vi "HFRR ADV v04.vi"() -> ()   [LabVIEW 2025] (continued)
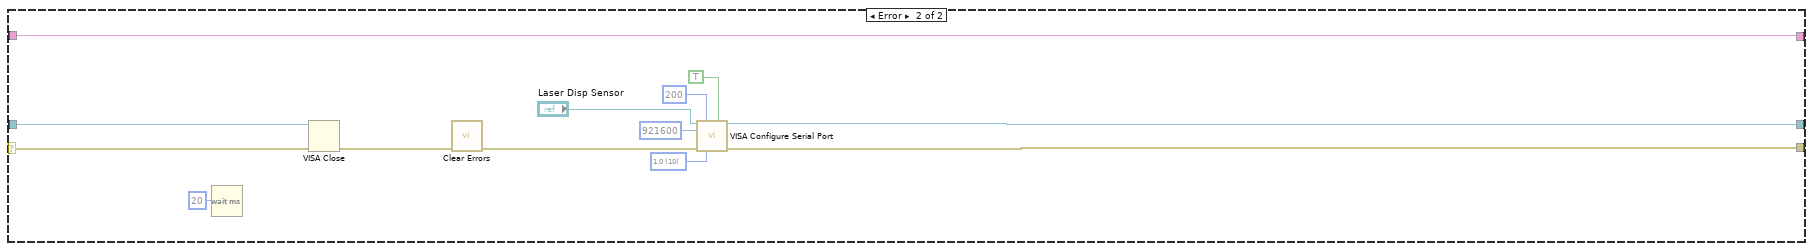
[diagram p11: hidden frame]
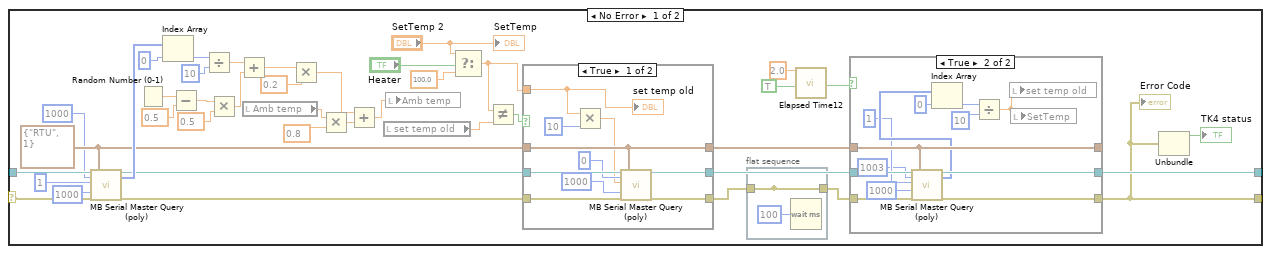
[diagram p13: hidden frame]
            n2851 = Concatenate Strings(w3863, w3862, w3864) -> (w3861:string)
            n2852 = Concatenate Strings(w3860, w3872, w3889, w3830) -> (w3836:string)
            n2853 = Concatenate Strings(w3860, w3871, w3882, w3830) -> (w3835:string)
            n2854 = Concatenate Strings(w3860, w3870, w3881, w3830) -> (w3834:string)
            n2855 = Concatenate Strings(w3860, w3869, w3874, w3830) -> (w3833:string)
            n2856 = Concatenate Strings(w3860, w3859, w3868, w3830) -> (w3832:string)
            n2857 = Concatenate Strings(w3860, w3858, w3861, "\"}" ("string")) -> (w3831:string)
            n2858 = Concatenate Strings(w3837, w3836, w3835, w3834, w3833, w3832, w3831, "]}" ("string")) -> (w3828:string)
            n2859 = local read "SEN.RUN HRS"() -> (w3795:dbl)
            n2860 = disable-structure shown="Disabled" {
              frame Disabled {
                n2861 = local read "state"() -> (w3914:string[])
                n2862 = Delete From Array(array=w3914, index=0) -> (array with subset deleted=w3912:string[])  [unwired: 1 in, 1 out]
                n2863 = for {
                  N: 6 -> [_]
                  tunnel: w3912 -> [w3925] mode=indexing
                  tunnel: [w3924] -> w3911 mode=indexing
                  n2864 = Equal?(x=w3925, y="Warning") -> (x = y?=w3921:bool)
                  n2865 = Equal?(x=w3925, y="Healthy") -> (x = y?=w3918:bool)
                  n2866 = Select(t="2" ("y"), s=w3921, f="3" ("y")) -> (s? t:f=w3916:string)
                  n2867 = Select(t="1" ("y"), s=w3918, f=w3916) -> (s? t:f=w3924:string)
                }
                "state1" <- w3911
              }
              frame Enabled {
              }
            }
            n2868 = stacked-sequence {
              tunnel: w3828 -> [w3936 _ _]
              tunnel: [_ _ w3952] -> _
              frame #0 {
                (unwired) FALSE ("convert eol (F)")
                w3938 = enum16{"start", "end", "current"}."start" ("pos mode (0:2)")
                n2869 = local read "Path"() -> (w3932:path)
                n2870 = Path To String(path=w3932) -> (string=w3944:string)
                n2871 = Concatenate Strings(w3944, "\\", "Sensor File Name") -> (w3945:string)
                n2872 = local write "standard output 2"(" ") -> ()
                n2873 = String To Path(string=w3945) -> (path=w3935:path)
                n2874 = call <vilib>:"Open_Create_Replace File.vi"("advisory dialog? (display:T)"=FALSE, "function (open:0)"=T22."create or replace", "file path"=w3935) -> ("error out"=w3948:errorcluster, "refnum"=w3947:refnum<file>)  [unwired: 5 in, 2 out]
                n2875 = Set File Position(refnum=w3947, from (0:start)=w3938, error in=w3948) -> (refnum out=w3928:refnum<file>, error out=w3927:errorcluster)  [unwired: 1 in]
                n2876 = Write to Binary File(file (use dialog)=w3928, data=" ", error in=w3927, 5:FALSE ("prepend array or string size? (T)")) -> (refnum out=w3939:refnum<file>, error out=w3940:errorcluster)  [unwired: 2 in, 1 out]
                n2877 = Set File Position(offset (in bytes) (0)=w3938, refnum=w3939, error in=w3940) -> (refnum out=w3931:refnum<file>, error out=w3930:errorcluster)  [unwired: 1 in]
                n2878 = Write to Binary File(file (use dialog)=w3931, data=w3936, error in=w3930, 5:FALSE ("prepend array or string size? (T)")) -> (error out=w3934:errorcluster)  [unwired: 2 in, 2 out]
                n2879 = flat-sequence {
                  tunnel: w3935 -> [w3950]
                  tunnel: w3934 -> [_]
                  frame #0 {
                    n2880 = call <vilib>:"Read Characters From File.vi"("file path (dialog if empty)"=w3950) -> ("character string"=→"Sensor Health JSON string":string)  [unwired: 5 in, 3 out]
                  }
                }
                "SinglePoint  2" <- w3936
              }
              frame #1 {
              }
              frame #2 {
                (unwired) "\"Stored\": true" ("string")
                n2881 = call <vilib>:"System Exec.vi"("run minimized? (F)"=TRUE, "wait until completion? (T)"=TRUE, "working directory"=path "C:/LAB-IQ-NXT", "command line"="C:\\LAB-IQ-NXT\\JPostH.bat") -> ("standard error"=→"Respose From Server 2":string, "standard output"=w3955:string)  [unwired: 4 in, 2 out]
                "standard output 2" <- w3955
                n2882 = Match Pattern(string=w3955, regular expression="JSONH Check String") -> (match substring=w3953:string, offset past match=w3952:i32)  [unwired: 1 in, 2 out]
                n2883 = Equal?(x=w3953, y="JSONH Check String") -> (x = y?=→"Upload \nConfirmed 2":bool)
              }
            }
            n2884 = Divide(x=w3795, y=3600.0 ("f")) -> (x/y=w3788:dbl)
            n2885 = local read "run time"() -> (w3845:string[])
            n2886 = Round To Nearest(number=w3788) -> (nearest integer value=w3787:dbl)
            n2887 = Number To Decimal String(number=w3787) -> (decimal integer string=w3786:string)  [unwired: 1 in]
            n2888 = Index Array(array="Sensor Information", index (col) #1=0 ("disabled index (col)"), index (col) #2=1 ("index (col)"), index (col) #3=2 ("index (col)"), index (col) #4=3 ("index (col)")) -> (element #1=→"Sensor name":string[], element #2=→"model num":string[], element #3=→"run time":string[], element #4=→"state":string[])  [unwired: 4 in]
            n2889 = Insert Into Array(array=w3845, index=1, new element #1=w3786, new element #2=w3786, new element #3=w3786, new element #4=w3786, new element #5=w3786, new element #6=w3786) -> (w3810:string[])
            "run" <- w3810
            n2890 = local read "out"() -> (w3792:string[])
            n2891 = local read "Sensor Information"() -> (w3812:string[][])
            n2892 = Replace Array Subset(array=w3812, new element #1=w3810, index (col) #1=2 ("disabled index (col)"), new element #2=w3792, index (col) #2=3 ("index (col)")) -> (w3811:string[][])  [unwired: 2 in]
            n2893 = local write "Sensor Information"(w3811) -> ()
          }
        }
        n2894 = case shown="True" w3759 {
          frame False {
          }
          frame True {
            n2895 = Equal?(x="FLAG", y=0.0) -> (x = y?=w3776:bool)
            n2896 = case shown="False" w3776 {
              frame False {
                n2897 = Get Date/Time In Seconds() -> (seconds since 1Jan1904=w3782:timestamp)
                n2898 = local read "START 2"() -> (w3780:dbl)
                n2899 = To Double Precision Float(number=w3782) -> (double precision float=w3781:dbl)
                n2900 = Subtract(x=w3781, y=w3780) -> (x-y=→"SENSOR TIME  2":dbl)
              }
              frame True {
                n2901 = Get Date/Time In Seconds() -> (seconds since 1Jan1904=w3784:timestamp)
                n2902 = To Double Precision Float(number=w3784) -> (double precision float=→"START 2":dbl)
                n2903 = local write "FLAG"(100.0 ("FLAG")) -> ()
              }
            }
          }
        }
        n2904 = disable-structure shown="Disabled" {
          disable-tunnel: w3762 -> [w3771 _]
          disable-tunnel: [w3770 _] -> w3761
          frame Disabled {
            n2905 = local read "Json St Flg"() -> (w3769:bool)
            n2906 = case shown="True" w3769 {
              tunnel: w3771 -> [w3772 w3774]
              tunnel: [w3772 w3773] -> w3770
              frame False {
              }
              frame True {
                n2907 = Increment(x=w3774) -> (x+1=w3773:dbl)
                "T cycle" <- w3773
                n2908 = local write "Json St Flg"(FALSE ("Json St Flg")) -> ()
              }
            }
          }
          frame Enabled {
          }
        }
        n2909 = local read "EXIT"() -> (w3756:bool)
      }
    }
    frame Enabled {
    }
  }
  n2910 = stacked-sequence {
    tunnel: [w4154] -> w16
    frame #0 {
      w4154 = FALSE ("Upload \nConfirmed")
      n2911 = local write "Upload \nConfirmed"(w4154) -> ()
      n2912 = local write "St Str"("") -> ()
    }
  }
  n2913 = disable-structure shown="Disabled" {
    disable-tunnel: w16 -> [w4155 _]
    frame Disabled {
      n2914 = case shown="True" {
        selector: _ -> [_ _]
        tunnel: w4155 -> [_ w4156]
        frame False {
        }
        frame True {
          n2915 = while {
            tunnel: [w4162] -> _
            tunnel: w4156 -> [_]
            i -> [w4162]
            stop <- w4159 stop-if-true
            n2916 = local read "Json End Flg"() -> (w4161:bool)
            n2917 = Wait (ms)(milliseconds to wait=u32 20 ("Refresh Rate (ms)")) -> ()  [unwired: 1 out]
            n2918 = local read "refresh flag"() -> (w4157:bool)
            n2919 = local read "RUN"() -> (w4158:bool)
            n2920 = And(x=w4158, y=w4157) -> (x .and. y?=w4160:bool)
            n2921 = Or(x=w4160, y=w4161) -> (x .or. y?=w4163:bool)
            "AR Led" <- w4163
            n2922 = case shown="True" w4163 {
              frame False {
              }
              frame True {
                w4180 = "\",\""
                n2923 = local read "UUID"() -> (w4178:string)
                n2924 = local write "refresh flag"(FALSE ("refresh flag")) -> ()
                n2925 = local read "time"() -> (w4167:dbl)
                n2926 = Multiply(x=w4167, y=60.0) -> (x*y=w4166:dbl)
                n2927 = Concatenate Strings("UUID\" : \"", w4178, "\"}") -> (w4181:string)
                n2928 = Number To Fractional String(number=w4166, width (-)=i16 10, precision (6)=i16 4) -> (F-format string=w4195:string)  [unwired: 1 in]
                n2929 = Concatenate Strings("{", "\"Time\":\"", w4195, w4180) -> (w4190:string)
                n2930 = stacked-sequence {
                  tunnel: w4180 -> [w4243 w4251 w4258 w4266 w4274 w4283 w4290]
                  tunnel: [w4244 _ _ _ _ _ _] -> w4194
                  tunnel: [_ w4252 _ _ _ _ _] -> w4193
                  tunnel: [_ _ w4259 _ _ _ _] -> w4192
                  tunnel: [_ _ _ w4268 _ _ _] -> w4191
                  tunnel: w4181 -> [_ _ _ _ _ _ w4301]
                  tunnel: [_ _ _ _ _ _ w4300] -> w4177
                  tunnel: [_ _ _ _ _ w4280 _] -> w4176
                  tunnel: [_ _ _ _ w4273 _ _] -> w4175
                  frame #0 {
                    n2931 = local read "NORMAL LOAD"() -> (w4242:dbl)
                    n2932 = Number To Fractional String(number=w4242, width (-)=i16 10, precision (6)=i16 4) -> (F-format string=w4245:string)  [unwired: 1 in]
                    n2933 = Concatenate Strings("NormalLoad\":\"", w4245, w4243) -> (w4244:string)
                  }
                  frame #1 {
                    n2934 = local read "Temp"() -> (w4250:dbl)
                    n2935 = Number To Fractional String(number=w4250, width (-)=i16 10, precision (6)=i16 4) -> (F-format string=w4253:string)  [unwired: 1 in]
                    n2936 = Concatenate Strings("Temperature\":\"", w4253, w4251) -> (w4252:string)
                  }
                  frame #2 {
                    n2937 = local read "cof"() -> (w4256:dbl)
                    n2938 = Number To Fractional String(number=w4256, width (-)=i16 10, precision (6)=i16 4) -> (F-format string=w4260:string)  [unwired: 1 in]
                    n2939 = Concatenate Strings("FrictionalForce\":\"", w4260, w4258) -> (w4259:string)
                  }
                  frame #3 {
                    n2940 = local read "Set Hz"() -> (w4264:dbl)
                    n2941 = Multiply(x=w4264, y=60.0) -> (x*y=w4263:dbl)
                    n2942 = Number To Fractional String(number=w4263, width (-)=i16 10, precision (6)=i16 4) -> (F-format string=w4269:string)  [unwired: 1 in]
                    n2943 = Concatenate Strings("Speed\":\"", w4269, w4266) -> (w4268:string)
                  }
                  frame #4 {
                    n2944 = local read "Stroke Ln"() -> (w4272:dbl)
                    n2945 = Number To Fractional String(number=w4272, width (-)=i16 10, precision (6)=i16 4) -> (F-format string=w4276:string)  [unwired: 1 in]
                    n2946 = Concatenate Strings("LinearDeformation\":\"", w4276, w4274) -> (w4273:string)
                  }
                  frame #5 {
                    n2947 = local read "AIR TEMP"() -> (w4279:dbl)
                    n2948 = local read "Json St Flg"() -> (w4281:bool)
                    n2949 = local read "Json End Flg"() -> (w4282:bool)
                    n2950 = Number To Fractional String(number=w4279, width (-)=i16 10, precision (6)=i16 4) -> (F-format string=w4285:string)  [unwired: 1 in]
                    n2951 = Concatenate Strings("Vibration\":\"", w4285, w4283) -> (w4280:string)
                    n2952 = And(x=w4281, y=w4282) -> ()  [unwired: 1 out]
                  }
                  frame #6 {
                    n2953 = local read "Json End Flg"() -> (w4289:bool)
                    n2954 = Get Date/Time In Seconds() -> (seconds since 1Jan1904=w4297:timestamp)
                    n2955 = local read "Json St Flg"() -> (w4288:bool)
                    n2956 = To Double Precision Float(number=w4297) -> (double precision float=w4296:dbl)
                    n2957 = Subtract(x=w4296, y=2082844800.0) -> (x-y=w4294:dbl)
                    n2958 = Number To Fractional String(number=w4294, width (-)=i16 12, precision (6)=i16 0) -> (F-format string=w4291:string)  [unwired: 1 in]
                    n2959 = case shown="True" w4289 {
                      tunnel: ["" w4304] -> w4298
                      tunnel: w4291 -> [_ w4305]
                      tunnel: w4290 -> [_ w4303]
                      frame False {
                      }
                      frame True {
                        n2960 = local write "Json End Flg"(FALSE ("Json St Flg")) -> ()
                        n2961 = Concatenate Strings("End\": \"", w4305, w4303) -> (w4304:string)
                      }
                    }
                    n2962 = case shown="True" w4288 {
                      tunnel: [w4308 w4311] -> w4299
                      tunnel: w4291 -> [_ w4312]
                      tunnel: w4290 -> [_ w4309]
                      frame False {
                        n2963 = local read "St Str"() -> (w4308:string)
                      }
                      frame True {
                        n2964 = Concatenate Strings("Start\":\"", w4312, w4309) -> (w4311:string)
                        "St Str" <- w4311
                        n2965 = local write "Json St Flg"(FALSE ("Json St Flg")) -> ()
                      }
                    }
                    n2966 = Concatenate Strings(w4299, w4298, w4301) -> (w4300:string)
                  }
                }
                n2967 = local read "FILE"() -> (w4169:string)
                n2968 = Concatenate Strings("\",\"OperatorID\":\"" ("string"), "Operator ID") -> (w4172:string)
                n2969 = Concatenate Strings("\",\"DatasetTitle\":\"" ("string"), w4169) -> (w4171:string)
                n2970 = Concatenate Strings("\",\"SerialNumber\":\"" ("string"), "Serial No") -> (w4201:string)
                n2971 = Concatenate Strings("\",\"ModelNumber\":\"" ("string"), "Model No") -> (w4200:string)
                n2972 = Concatenate Strings(w4201, w4200) -> (w4183:string)
                n2973 = Concatenate Strings("{\"SecretKey\":\"", "Secret Key", w4183, w4172, w4171, "\",\"Samples\":[") -> (w4188:string)
                n2974 = Concatenate Strings(w4190, w4194, w4193, w4192, w4191, w4175, w4176, w4177) -> (w4189:string)
                n2975 = Concatenate Strings(w4188, w4189, "]}") -> (w4187:string)
                n2976 = stacked-sequence {
                  tunnel: w4187 -> [w4216 _ _]
                  tunnel: [_ _ w4233] -> _
                  frame #0 {
                    (unwired) FALSE ("convert eol (F)")
                    w4218 = enum16{"start", "end", "current"}."start" ("pos mode (0:2)")
                    n2977 = Path To String(path="Path") -> (string=w4224:string)
                    n2978 = Concatenate Strings(w4224, "\\", "Data File Name") -> (w4226:string)
                    n2979 = local write "standard output"(" ") -> ()
                    n2980 = String To Path(string=w4226) -> (path=w4215:path)
                    n2981 = call <vilib>:"Open_Create_Replace File.vi"("advisory dialog? (display:T)"=FALSE, "function (open:0)"=T22."create or replace", "file path"=w4215) -> ("error out"=w4229:errorcluster, "refnum"=w4228:refnum<file>)  [unwired: 5 in, 2 out]
                    n2982 = Set File Position(refnum=w4228, from (0:start)=w4218, error in=w4229) -> (refnum out=w4209:refnum<file>, error out=w4208:errorcluster)  [unwired: 1 in]
                    n2983 = Write to Binary File(file (use dialog)=w4209, data=" ", error in=w4208, 5:FALSE ("prepend array or string size? (T)")) -> (refnum out=w4219:refnum<file>, error out=w4220:errorcluster)  [unwired: 2 in, 1 out]
                    n2984 = Set File Position(offset (in bytes) (0)=w4218, refnum=w4219, error in=w4220) -> (refnum out=w4212:refnum<file>, error out=w4211:errorcluster)  [unwired: 1 in]
                    n2985 = Write to Binary File(file (use dialog)=w4212, data=w4216, error in=w4211, 5:FALSE ("prepend array or string size? (T)")) -> (error out=w4214:errorcluster)  [unwired: 2 in, 2 out]
                    n2986 = flat-sequence {
                      tunnel: w4215 -> [w4231]
                      tunnel: w4214 -> [_]
                      frame #0 {
                        n2987 = call <vilib>:"Read Characters From File.vi"("file path (dialog if empty)"=w4231) -> ("character string"=→"JSON string":string)  [unwired: 5 in, 3 out]
                      }
                    }
                    "SinglePoint" <- w4216
                  }
                  frame #1 {
                  }
                  frame #2 {
                    (unwired) "\"Stored\": true" ("string")
                    n2988 = call <vilib>:"System Exec.vi"("run minimized? (F)"=TRUE, "wait until completion? (T)"=TRUE, "working directory"=path "C:/LAB-IQ-NXT", "command line"="C:\\LAB-IQ-NXT\\JPost.bat") -> ("standard error"=→"Respose From Server":string, "standard output"=w4236:string)  [unwired: 4 in, 2 out]
                    "standard output" <- w4236
                    n2989 = Match Pattern(string=w4236, regular expression="JSON Check String") -> (match substring=w4234:string, offset past match=w4233:i32)  [unwired: 1 in, 2 out]
                    n2990 = Equal?(x=w4234, y="JSON Check String") -> (x = y?=→"Upload \nConfirmed":bool)
                  }
                }
              }
            }
            n2991 = local read "EXIT"() -> (w4159:bool)
          }
        }
      }
    }
    frame Enabled {
    }
  }
  n2992 = disable-structure shown="Disabled" {
    disable-tunnel: w15 -> [w4319 _]
    frame Disabled {
      n2993 = while {
        shift-right: [w4327] -> w4315
        shift-left: _ -> [w4328]
        shift-right: [w4325] -> w4316
        shift-left: errorcluster {"status"=TRUE, "code"=0, "source"="Init"} ("error out") -> [w4326]
        shift-right: [w4323] -> _
        shift-left: "" -> [w4324]
        tunnel: [w4321] -> _
        tunnel: w4319 -> [_]
        i -> [w4321]
        stop <- w4320 stop-if-true
        n2994 = flat-sequence {
          tunnel: [w4329] -> w4322
          frame #0 {
            n2995 = Wait (ms)(milliseconds to wait=10.0 ("Delay")) -> (millisecond timer value=w4329:u32)
          }
        }
        n2996 = case shown="No Error" w4326 {
          selector: w4326 -> [w4362 w4484]
          tunnel: [w4344 w4486] -> w4327
          tunnel: [w4343 w4485] -> w4325
          tunnel: w4328 -> [w4363 w4478]
          tunnel: w4324 -> [w4342 w4477]
          tunnel: [w4341 w4477] -> w4323
          tunnel: w4322 -> [_ _]
          frame No Error {
            n2997 = Concatenate Strings("COMMAND", "\r", "\n") -> (w4353:string)
            n2998 = case shown="True" "Measure" {
              tunnel: w4363 -> [w4389 w4396]
              tunnel: w4362 -> [w4388 w4395]
              tunnel: [w4389 w4394] -> w4361
              tunnel: [w4388 w4393] -> w4340
              tunnel: w4353 -> [_ w4392]
              frame False {
              }
              frame True {
                n2999 = VISA Write(VISA resource name=w4396, write buffer=w4392, error in (no error)=w4395) -> (VISA resource name out=w4394:refnum<visa-resource-name>, error out=w4393:errorcluster)  [unwired: 1 out]
                n3000 = local write "Read String"("") -> ()
                n3001 = local write "Measure"(FALSE) -> ()
              }
            }
            n3002 = property class="Instr"(reference=w4361, error in=w4340) -> (reference out=w4360:refnum<visa-resource-name>, error out=w4359:errorcluster, "Serial Settings:Number of Bytes at Serial Port"=w4358:u32)
            n3003 = Greater?(x=w4358, y=u32 100) -> (0:w4356:bool)
            n3004 = case shown="True" w4356 {
              tunnel: w4360 -> [w4399 w4424]
              tunnel: w4359 -> [w4398 w4423]
              tunnel: w4358 -> [_ w4422]
              tunnel: [w4399 w4421] -> w4346
              tunnel: [w4398 w4420] -> w4345
              tunnel: w4342 -> [w4397 w4419]
              tunnel: [w4397 ""] -> w4341
              frame False {
              }
              frame True {
                w4409 = u32 6 ("y")
                # "Page 84 of \nmanual"
                n3005 = VISA Read(VISA resource name=w4424, byte count=w4422, error in (no error)=w4423) -> (VISA resource name out=w4421:refnum<visa-resource-name>, read buffer=w4417:string, error out=w4420:errorcluster)  [unwired: 1 out]
                n3006 = while {
                  tunnel: w4417 -> [w4473]
                  tunnel: [w4469] -> w4411 mode=indexing
                  tunnel: [w4463] -> w4415 mode=indexing
                  tunnel: [w4461] -> _
                  i -> [w4461]
                  stop <- w4466 stop-if-true
                  n3007 = String Subset(string=w4473, offset (0)=w4461) -> (substring=w4468:string)  [unwired: 1 in]
                  n3008 = String To Byte Array(string=w4468) -> (unsigned byte array=w4472:u8[])
                  n3009 = String Length(string=w4468) -> (length=w4467:i32)
                  n3010 = Index Array(array=w4472) -> (element=w4471:u8)  [unwired: 1 in]
                  n3011 = Equal To 0?(x=w4467) -> (x = 0?=w4466:bool)
                  n3012 = Number To Boolean Array(number=w4471) -> (Boolean array=w4465:bool[])
                  n3013 = Reverse 1D Array(array=w4465) -> (reversed array=w4464:bool[])
                  n3014 = And(x=w4465, y=bool[] [FALSE, FALSE, FALSE, FALSE, FALSE, FALSE, TRUE, TRUE] ("Boolean array")) -> (x .and. y?=w4469:bool[])
                  n3015 = And(x=w4464, y=bool[] [FALSE, FALSE, TRUE, TRUE, TRUE, TRUE, TRUE, TRUE] ("Boolean array")) -> (x .and. y?=w4463:bool[])
                }
                n3016 = Concatenate Strings(w4419, w4417) -> (→"Read String":string)
                n3017 = while {
                  tunnel: w4411 -> [w4460] mode=indexing
                  tunnel: [w4456] -> w4414
                  i -> [w4456]
                  stop <- w4457 stop-if-true
                  n3018 = Search 1D Array(1D array=w4460, element=TRUE) -> (index of element=w4458:i32)  [unwired: 1 in]
                  n3019 = Less Than 0?(x=w4458) -> (x < 0?=w4457:bool)
                }
                n3020 = Delete From Array(array=w4415, length=w4414, index (row)=0) -> (array with subset deleted=w4410:bool[][])  [unwired: 1 in, 1 out]
                n3021 = Array Size(array=w4410) -> (size(s)=w4412:i32[])
                n3022 = Index Array(array=w4412) -> (element=w4404:i32)  [unwired: 1 in]
                n3023 = Greater?(x=w4404, y=w4409) -> (0:w4407:bool)
                n3024 = Subtract(x=w4404, y=w4409) -> (x-y=w4408:u32)
                n3025 = Select(t=w4408, s=w4407, f=u32 0) -> (s? t:f=w4405:u32)
                n3026 = while {
                  tunnel: w4410 -> [w4443]
                  tunnel: [w4445] -> w4403 mode=indexing
                  tunnel: w4405 -> [w4427]
                  i -> [w4444]
                  stop <- w4442 stop-if-true
                  w4434 = 6 ("index")
                  w4433 = 2 ("length")
                  # "Page 65 of \nmanual"
                  n3027 = Multiply(x=u32 3 ("y"), y=w4444) -> (x*y=w4441:u32)
                  n3028 = Divide(x=u32 102 ("y"), y=u32 65520) -> (x/y=w4451:dbl)
                  n3029 = Greater Or Equal?(x=w4441, y=w4427) -> (x >= y?=w4442:bool)
                  n3030 = Index Array(array=w4443, index (row) #1=w4441) -> (element #1=w4439:bool[], element #2=w4438:bool[], element #3=w4437:bool[])  [unwired: 5 in]
                  n3031 = Reverse 1D Array(array=w4439) -> (reversed array=w4432:bool[])
                  n3032 = Reverse 1D Array(array=w4438) -> (reversed array=w4436:bool[])
                  n3033 = Reverse 1D Array(array=w4437) -> (reversed array=w4435:bool[])
                  n3034 = Delete From Array(array=w4432, length=w4433, index=w4434) -> (array with subset deleted=w4428:bool[])  [unwired: 1 out]
                  n3035 = Delete From Array(array=w4436, length=w4433, index=w4434) -> (array with subset deleted=w4429:bool[])  [unwired: 1 out]
                  n3036 = Delete From Array(array=w4435, length=w4433, index=w4434) -> (array with subset deleted=w4430:bool[])  [unwired: 1 out]
                  n3037 = Insert Into Array(array=bool[] [] ("Boolean array"), new element #1=w4428, new element #2=w4429, new element #3=w4430) -> (w4431:bool[])  [unwired: 1 in]
                  n3038 = Boolean Array To Number(Boolean array=w4431) -> (number=w4440:u32)
                  n3039 = Multiply(x=w4451, y=w4440) -> (x*y=w4450:dbl)
                  n3040 = Decrement(x=w4450) -> (x-1=w4449:dbl)
                  n3041 = Divide(x=w4449, y=u32 100) -> (x/y=w4447:dbl)
                  n3042 = Multiply(x=w4447, y=u32 10) -> (x*y=w4445:dbl)
                }
                n3043 = Delete From Array(array=w4403) -> (array with subset deleted=w4402:dbl[])  [unwired: 2 in, 1 out]
                "Waveform Graph 5" <- w4402
                "Waveform Chart 3" <- w4402
                n3044 = call-poly <vilib>:"Mean.vi"("X"=w4402) -> ("mean"=w4401:dbl)  [unwired: 1 out]
                "Measure_LDS" <- w4401
                n3045 = case shown="True" "Zero 4" {
                  tunnel: w4401 -> [_ w4426]
                  frame False {
                  }
                  frame True {
                    n3046 = local write "Zero 4"(FALSE ("Zero 4")) -> ()
                    "z_measure" <- w4426
                  }
                }
              }
            }
            n3047 = local read "Measure_LDS"() -> (w4336:dbl)
            n3048 = local read "Disp (mm)"() -> (w4335:dbl)
            n3049 = local read "Boolean 7"() -> (w4334:bool)
            n3050 = local read "Boolean 8"() -> (w4333:bool)
            n3051 = case shown="True" "Boolean 8" {
              tunnel: w4335 -> [_ w4366]
              tunnel: w4336 -> [_ w4365]
              frame False {
              }
              frame True {
                n3052 = local read "Captured Values 2"() -> (w4369:dbl[][])
                n3053 = Build Array(w4366, w4365) -> (w4364:dbl[])
                n3054 = Build Array (concatenate)(w4369, w4364) -> (w4367:dbl[][])
                n3055 = local write "Captured Values 2"(w4367) -> ()
                n3056 = local write "Boolean 8"(FALSE ("Boolean 8")) -> ()
              }
            }
            n3057 = call "Build XY Graph"("Enable"=w4333, "Reset"=w4334, "Y Input"=w4336, "X Input"=w4335) -> ("XY Graph"=→"?":cluster{"Y":dbl[], "Y":dbl[]}[])  [unwired: 6 in, 1 out]
            n3058 = case shown="True" "Boolean 9" {
              frame False {
              }
              frame True {
                n3059 = local read "Captured Values 2"() -> (w4371:dbl[][])
                n3060 = Index Array(array=w4371, index (col) #1=0 ("disabled index (col)"), index (col) #2=1 ("index (col)")) -> (element #1=w4374:dbl[], element #2=w4373:dbl[])  [unwired: 2 in]
                n3061 = call <vilib>:"Linear Fit.vi"("Y"=w4374, "X"=w4373) -> ("slope"=→"Slope":dbl, "intercept"=→"Intercept":dbl)  [unwired: 9 in, 3 out]
                n3062 = local write "Boolean 9"(FALSE ("Boolean 9")) -> ()
              }
            }
            n3063 = case shown="True" "Boolean 7" {
              frame False {
              }
              frame True {
                n3064 = local write "Captured Values 2"(dbl[][] [] ("Captured Values")) -> ()
                n3065 = local write "Boolean 7"(FALSE ("Boolean 7")) -> ()
              }
            }
            n3066 = Concatenate Strings("COMMAND 2", "\r", "\n") -> (w4348:string)
            n3067 = case shown="True" "Measure 2" {
              tunnel: w4346 -> [w4381 w4387]
              tunnel: w4345 -> [w4380 w4386]
              tunnel: [w4381 w4385] -> w4344
              tunnel: [w4380 w4384] -> w4343
              tunnel: w4348 -> [_ w4383]
              frame False {
              }
              frame True {
                n3068 = local write "Measure 2"(FALSE ("WRITE")) -> ()
                n3069 = VISA Write(VISA resource name=w4387, write buffer=w4383, error in (no error)=w4386) -> (VISA resource name out=w4385:refnum<visa-resource-name>, error out=w4384:errorcluster)  [unwired: 1 out]
              }
            }
          }
          frame Error {
            w4476 = u16 10 items=["1.0"=10, "1.5"=15, "2.0"=20] ("stop bits (10: 1 bit)")
            n3070 = Wait (ms)(milliseconds to wait=u32 20) -> ()  [unwired: 1 out]
            n3071 = VISA Close(VISA resource name=w4478, error in (no error)=w4484) -> (error out=w4483:errorcluster)
            n3072 = call <vilib>:"Clear Errors.vi"("error in (no error)"=w4483) -> ("error out"=w4482:errorcluster)  [unwired: 5 in, 1 out]
            n3073 = call-poly "VISA Configure Serial Port"("VISA resource name"="Laser Disp Sensor", "timeout (10sec)"=u32 200, "Enable Termination\nChar (T)"=TRUE ("Enable Termination\nChar (T)"), "baud rate (9600)"=u32 921600, "error in (no error)"=w4482, "stop bits (10: 1 bit)"=w4476) -> ("VISA resource name out"=w4486:refnum<visa-resource-name>, "error out"=w4485:errorcluster)  [unwired: 8 in]
          }
        }
        n3074 = local read "EXIT"() -> (w4320:bool)
      }
      n3075 = VISA Close(VISA resource name=w4315, error in (no error)=w4316) -> (error out=w4314:errorcluster)
      n3076 = call <vilib>:"Clear Errors.vi"("error in (no error)"=w4314) -> ()  [unwired: 5 in, 2 out]
    }
    frame Enabled {
    }
  }
  n3077 = disable-structure shown="Disabled" {
    disable-tunnel: w15 -> [w4491 _]
    frame Disabled {
      n3078 = while {
        tunnel: [w4498] -> _
        shift-right: [w4495] -> w4488
        shift-left: _ -> [w4497]
        shift-right: [w4496] -> w4489
        shift-left: errorcluster {"status"=TRUE, "code"=0, "source"="Init"} ("error out") -> [w4494]
        tunnel: w4491 -> [_]
        i -> [w4498]
        stop <- w4492 stop-if-true
        n3079 = flat-sequence {
          tunnel: w4494 -> [w4589]
          tunnel: [w4589] -> w4493
          frame #0 {
            n3080 = Wait (ms)(milliseconds to wait=u32 50) -> ()  [unwired: 1 out]
          }
        }
        n3081 = case shown="Error" w4493 {
          selector: w4493 -> [w4539 w4582]
          tunnel: w4497 -> [w4538 w4581]
          tunnel: [w4505 w4572] -> w4496
          tunnel: [w4506 w4580] -> w4495
          frame No Error {
            w4532 = T23 {"Mode"=enum."RTU", "Slave Address"=1} ("Serial Parameters")
            n3082 = call-poly <vilib>:"MB Serial Master Query (poly).vi"("VISA resource name"=w4538, "Starting Address"=i16 1000, "Quantity"=u16 1, "Timeout"=u32 1000, "error in"=w4539, "Serial Parameters"=w4532) -> ("VISA resource name out"=w4533:refnum<visa-resource-name>, "Input Registers"=w4535:u16[], "error out"=w4531:errorcluster)  [unwired: 10 in, 1 out]
            n3083 = Random Number (0-1)() -> (number: 0 to 1=w4520:dbl)
            n3084 = Index Array(array=w4535, index=0) -> (element=w4530:u16)
            n3085 = Subtract(x=w4520, y=0.5) -> (x-y=w4519:dbl)
            n3086 = Divide(x=w4530, y=10 ("index")) -> (x/y=w4524:dbl)
            n3087 = Multiply(x=w4519, y=0.5) -> (x*y=w4518:dbl)
            n3088 = Add(x=w4524, y=w4518) -> (x+y=w4523:dbl)
            n3089 = local read "Amb temp"() -> (w4507:dbl)
            n3090 = Multiply(x=w4523, y=0.2) -> (x*y=w4527:dbl)
            n3091 = Multiply(x=w4507, y=0.8) -> (x*y=w4525:dbl)
            n3092 = Add(x=w4527, y=w4525) -> (x+y=w4508:dbl)
            n3093 = local read "set temp old"() -> (w4502:dbl)
            n3094 = local write "Amb temp"(w4508) -> ()
            n3095 = Select(t="SetTemp 2", s="Heater", f=100.0) -> (s? t:f=w4503:dbl)
            n3096 = Not Equal?(x=w4503, y=w4502) -> (x != y?=w4501:bool)
            n3097 = case shown="True" w4501 {
              tunnel: w4533 -> [w4567 w4569]
              tunnel: [w4566 w4569] -> w4513
              tunnel: w4531 -> [w4565 w4568]
              tunnel: [w4564 w4568] -> w4511
              tunnel: w4503 -> [w4559 _]
              tunnel: w4532 -> [w4561 w4570]
              tunnel: [w4561 w4570] -> w4514
              frame True {
                n3098 = Multiply(x=w4559, y=10 ("index")) -> (x*y=w4558:dbl)
                n3099 = call-poly <vilib>:"MB Serial Master Query (poly).vi"("VISA resource name"=w4567, "Address"=u16 0, "Holding Register"=w4558, "Timeout"=u32 1000, "error in"=w4565, "Serial Parameters"=w4561) -> ("VISA resource name out"=w4566:refnum<visa-resource-name>, "error out"=w4564:errorcluster)  [unwired: 11 in, 1 out]
                "set temp old" <- w4559
              }
              frame False {
              }
            }
            n3100 = flat-sequence {
              tunnel: [w4540] -> _
              tunnel: [w4540] -> w4510
              tunnel: w4511 -> [w4540]
              frame #0 {
                n3101 = Wait (ms)(milliseconds to wait=u32 100) -> ()  [unwired: 1 out]
              }
            }
            n3102 = call "Elapsed Time12"("Time Target (s)"=2.0, "Auto Reset"=TRUE) -> ("Time has Elapsed"=w4515:bool)  [unwired: 10 in, 7 out]
            n3103 = case shown="True" w4515 {
              tunnel: w4514 -> [w4544 w4557]
              tunnel: [w4544 w4557] -> _
              tunnel: [w4543 w4555] -> w4506
              tunnel: w4513 -> [w4543 w4556]
              tunnel: [w4542 w4553] -> w4505
              tunnel: w4510 -> [w4542 w4554]
              frame False {
              }
              frame True {
                n3104 = call-poly <vilib>:"MB Serial Master Query (poly).vi"("VISA resource name"=w4556, "Starting Address"=i16 1003 ("Addr"), "Quantity"=u16 1, "Timeout"=u32 1000, "error in"=w4554, "Serial Parameters"=w4557) -> ("VISA resource name out"=w4555:refnum<visa-resource-name>, "Input Registers"=w4550:u16[], "error out"=w4553:errorcluster)  [unwired: 10 in, 1 out]
                n3105 = Index Array(array=w4550, index=0) -> (element=w4549:u16)
                n3106 = Divide(x=w4549, y=u16 10) -> (x/y=w4545:dbl)
                n3107 = local write "set temp old"(w4545) -> ()
                n3108 = local write "SetTemp"(w4545) -> ()
              }
            }
            "Error Code" <- w4505
            n3109 = Unbundle(w4505) -> ("status"=→"TK4 status":bool)  [unwired: 2 out]
            "SetTemp" <- "SetTemp 2"
          }
          frame Error {
            w4584 = u16 0 items=["None", "Odd", "Even", "Mark", "Space"] ("Parity")
            w4585 = u16 0 items=["None", "XON/XOFF", "RTS/CTS", "XON/XOFF & RTS/CTS", "DTR/DSR", "XON/XOFF & DTR/DSR"] ("Flow Control")
            n3110 = VISA Clear(VISA resource name=w4581, error in (no error)=w4582) -> (VISA resource name out=w4575:refnum<visa-resource-name>, error out=w4573:errorcluster)
            n3111 = VISA Close(VISA resource name=w4575, error in (no error)=w4573) -> (error out=w4574:errorcluster)
            n3112 = call <vilib>:"Clear Errors.vi"("error in (no error)"=w4574) -> ("error out"=w4583:errorcluster)  [unwired: 5 in, 1 out]
            n3113 = Unbundle By Name(T23 {"Mode"=enum."RTU", "Slave Address"=1} ("input cluster")) -> ("Mode"=w4586:enum16{"RTU", "ASCII"})
            n3114 = call <vilib>:"MB Serial Init.vi"("Timeout"=u32 100, "Flow Control"=w4585, "Mode"=w4586, "error in (no error)"=w4583, "Parity"=w4584, "Baud Rate"=u32 9600, "VISA resource name"="Lubrication System COM Port :") -> ("error out"=w4572:errorcluster, "VISA resource name out"=w4580:refnum<visa-resource-name>)  [unwired: 3 in]
            n3115 = local write "set temp old"(0.0 ("set temp old")) -> ()
            n3116 = Unbundle(w4572) -> ("status"=w4571:bool)  [unwired: 2 out]
            n3117 = case shown="True" w4571 {
              selector: w4571 -> [_ w4588]
              frame False {
              }
              frame True {
                n3118 = local write "TK4 status"(w4588) -> ()
              }
            }
          }
        }
        n3119 = local read "EXIT"() -> (w4492:bool)
      }
      n3120 = VISA Close(VISA resource name=w4488, error in (no error)=w4489) -> (error out=w4487:errorcluster)
      n3121 = call <vilib>:"Clear Errors.vi"("error in (no error)"=w4487) -> ()  [unwired: 5 in, 2 out]
    }
    frame Enabled {
    }
  }
  "file count" <- 0 ("file count")
